vi "encodeExt.vi"(2 "ByteArray":u8[](array[numeric]) format="%.0x", 3 "Type":i8) -> (1 "MessagePack":u8[](array[numeric]) format="%.0x")   [LabVIEW 2015, in "MsgPack.lvlib"]
uses:
  MsgPack.lvlib
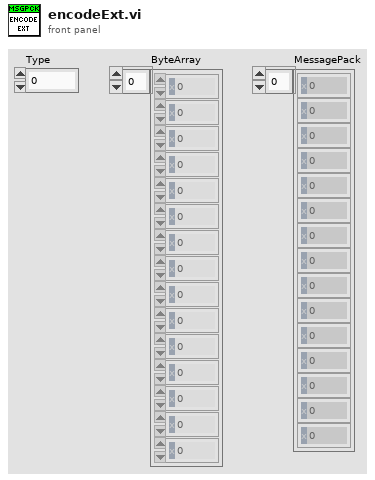
[diagram p1: front panel]
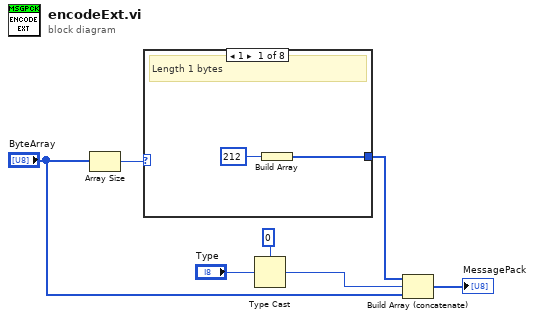
[diagram p0: block diagram]
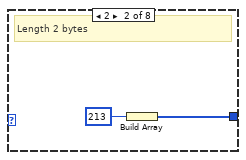
[diagram p2: hidden frame]
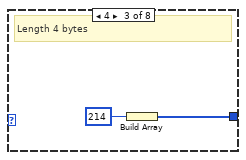
[diagram p3: hidden frame]
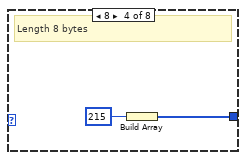
[diagram p4: hidden frame]
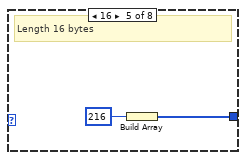
[diagram p5: hidden frame]
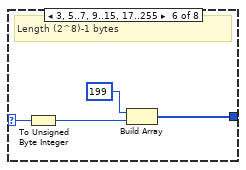
[diagram p6: hidden frame]
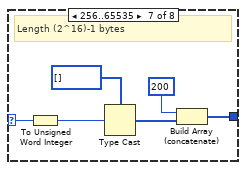
[diagram p7: hidden frame]
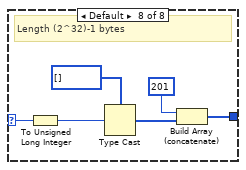
[diagram p8: hidden frame]
diagram:
  n1 = Array Size(array="ByteArray") -> (size(s)=w5:i32)
  n2 = case shown="1" w5 {
    selector: w5 -> [_ _ _ _ _ w19 w25 w31]
    tunnel: [w8 w10 w12 w14 w16 w20 w26 w32] -> w6
    frame 1 {
      # "Length 1 bytes"
      n3 = Build Array(u8 212) -> (w8:u8[])
    }
    frame 2 {
      # "Length 2 bytes"
      n4 = Build Array(u8 213) -> (w10:u8[])
    }
    frame 4 {
      # "Length 4 bytes"
      n5 = Build Array(u8 214) -> (w12:u8[])
    }
    frame 8 {
      # "Length 8 bytes"
      n6 = Build Array(u8 215) -> (w14:u8[])
    }
    frame 16 {
      # "Length 16 bytes"
      n7 = Build Array(u8 216) -> (w16:u8[])
    }
    frame 3, 5..7, 9..15, 17..255 {
      # "Length (2^8)-1 bytes"
      n8 = To Unsigned Byte Integer(number=w19) -> (unsigned 8bit integer=w18:u8)
      n9 = Build Array(u8 199, w18) -> (w20:u8[])
    }
    frame 256..65535 {
      # "Length (2^16)-1 bytes"
      n10 = To Unsigned Word Integer(number=w25) -> (unsigned 16bit integer=w24:u16)
      n11 = Type Cast(type=u8[] [] ("appended array"), x=w24) -> (*(type *) &x=w22:u8[])
      n12 = Build Array (concatenate)(u8 200, w22) -> (w26:u8[])
    }
    frame Default {
      # "Length (2^32)-1 bytes"
      n13 = To Unsigned Long Integer(number=w31) -> (unsigned 32bit integer=w30:u32)
      n14 = Type Cast(type=u8[] [] ("appended array"), x=w30) -> (*(type *) &x=w28:u8[])
      n15 = Build Array (concatenate)(u8 201, w28) -> (w32:u8[])
    }
  }
  n16 = Type Cast(type=u8 0, x="Type") -> (*(type *) &x=w2:u8)
  n17 = Build Array (concatenate)(w6, w2, "ByteArray") -> (→"MessagePack":u8[])
